vi "TSCAN_GetSignalValue.vi"(4 "ALLSignalName":string[][](array[string]), 6 "ALLMessage":string[](array[string]), 7 "ALLID":i32[](array[numeric]) format="%x", 8 "簇":T1, 11 "path":path) -> (0 "array":string[](array[string]), 1 "Element index":i32, 2 "SigValue":dbl[](array[numeric]), 3 "path out":path, 5 "return":i32[](array[numeric]))   [LabVIEW 2014]
doc: "获取 can 信号值\nObtain the CAN signal value"
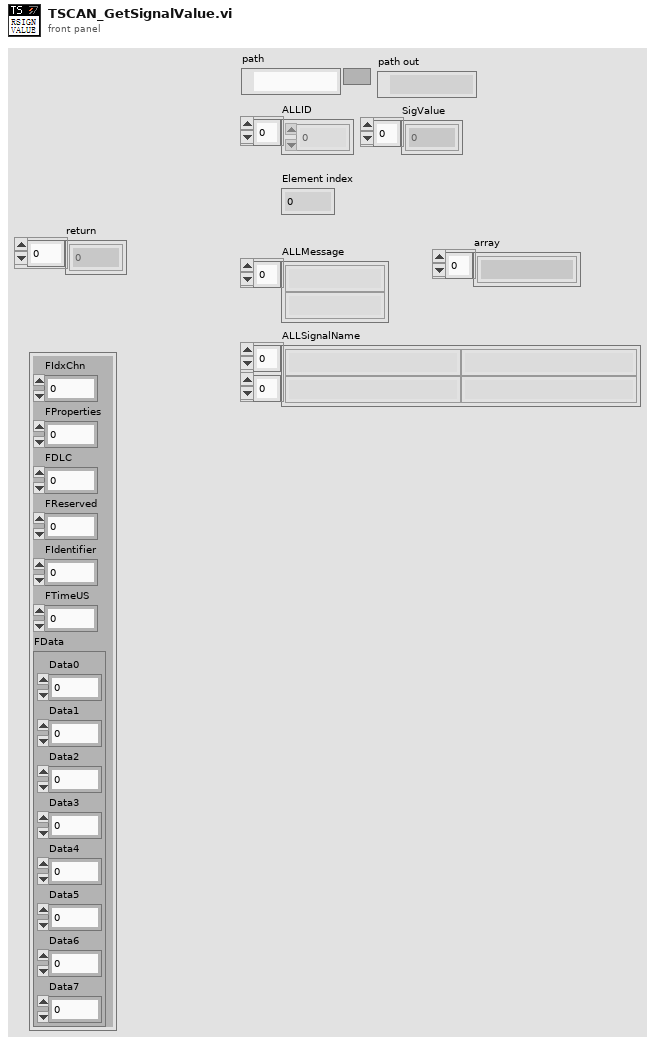
[diagram p1: front panel]
types:
  T1 = cluster{"FIdxChn":u8, "FProperties":u8, "FDLC":u8, "FReserved":u8, "FIdentifier":i32, "FTimeUS":u64, "FData":cluster{"Data0":u8, "Data1":u8, "Data2":u8, "Data3":u8, "Data4":u8, "Data5":u8, "Data6":u8, "Data7":u8}}
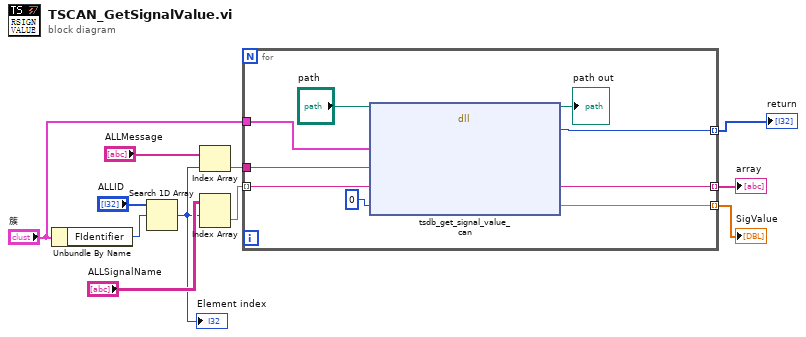
[diagram p0: block diagram]
diagram:
  n1 = Unbundle By Name("簇") -> ("FIdentifier"=w9:i32)
  n2 = Search 1D Array(1D array="ALLID", element=w9) -> (index of element=w5:i32)  [unwired: 1 in]
  "Element index" <- w5
  n3 = Index Array(array="ALLMessage", index=w5) -> (element=w7:string)
  n4 = Index Array(array="ALLSignalName", index (row)=w5) -> (element=w4:string[])  [unwired: 1 in]
  n5 = for {
    tunnel: "簇" -> [w20]
    tunnel: w7 -> [w19]
    tunnel: w4 -> [w15] mode=indexing
    tunnel: [w14] -> w3 mode=indexing
    tunnel: [w13] -> w2 mode=indexing
    tunnel: [w12] -> w1 mode=indexing
    n6 = dll-call lib="D:/Program Files (x86)/TOSUN/TSMaster/bin/TSMaster.dll" fn="tsdb_get_signal_value_can"(path in="path", "CANObJ"=w20, "Message"=w19, "Signal"=w15, "SigValue"=0) -> (path out=→"path out":path, "tsdb_get_signal_value_can"=w12:i32, "Signal"=w13:string, "SigValue"=w14:dbl)  [unwired: 4 in, 1 out]
  }
  "SigValue" <- w3
  "array" <- w2
  "return" <- w1
